vi "AlliGator Compute Pixel Phasor Array v3.vi"(6 "e^j w t_i Vector":csg[](array[numeric]), 7 "Time-Gated Reference Decay":cluster{"t Array":dbl[], "I Array":dbl[]}, 8 "Error In":errorcluster, 9 "t Array":sgl[](array[numeric]), 10 "Gate Images Stack (NxVxH)":sgl[][][](array[numeric]), 11 "Sum Image (V x H)":sgl[][](array[numeric])) -> (0 "Error Out":errorcluster, 1 "# Invalid Phasors":i32, 3 "Pixel Phasors Array (V x H)":csg[][](array[numeric]) format="%_3e", 4 "CPU (s)":dbl)   [LabVIEW 2021, in "AlliGator Phasor Plot.lvlib"]
doc: "Computes the phasor of all pixels using any user-selected decay pre-processing options."
uses:
  AlliGator Phasor Plot.lvlib
  AlliGator Settings List.ctl
  AlliGator Abort.vi
  <vilib>/Utility/error.llb/Error Cluster From Error Code.vi
  <vilib>/ErrorRing/Error Ring.xnode
  Time/Time.lvlib
  Phasor/Phasor.lvlib
  Graphs/XY Graph/XY Graph Add-Ons.lvlib
  AlliGator Decay Preprocessing.lvlib
  AlliGator Globals, Variables & Constants.lvlib
  AlliGator Settings.lvlib
  Error/Error.lvlib
  Utilities/Utilities.lvlib
panel:
  out "Local Error":errorcluster
  # "see the AlliGator License on the block diagram (Ctrl+E or Window:Show Block Diagram)"
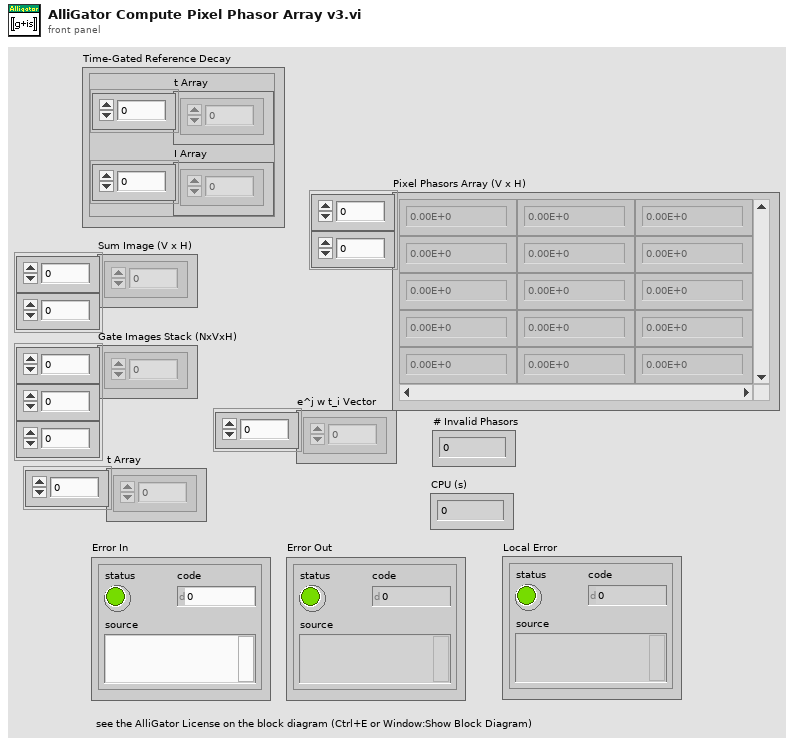
[diagram p1: front panel]
types:
  T1 = typedef "AlliGator Settings.lvlib/AlliGator Settings List.ctl" = enum16{"GUI:Visible Settings Tab", "GUI:Last Run Version", "Source Image:Use Image Histogram for Contrast", "Source Image:Low Count Pixels Rejection Options", "Source Image:High Count Pixels Rejection Options", "Source Image:Use Image Brightness", "Source Image:Blend Overlay with Image Background", "Source Image:Use Fixed ROI Diameter", "Source Image:ROI Diameter", "Source Image:ROI Center Color", "Source Image:Peak Threshold", "Source Image:Intensity Threshold", "Source Image:Image Binning Options", "Source Image:Image Smoothing Options", "Source Image:Image Histogram Active", "Source Image:Invert Binary Mask", "Source Image:Hot Pixel Removal", "Source Image:Overlay Analyzed ROI Center", "Source Image:Auto-Adjust Contrast", "Source Image:Histogram Lower Percentile", "Source Image:Histogram Upper Percentile", "Source Image:Save Source Image", "Source Image:Scale Bar Options", "Source Image:Image Resolution (Pixel Size)", "Source Image:Flatfield Correction", "Source Image:Show Dead Left Columns Correction", "Source Image:Dead Left Columns Correction", "Source Image:Image Pre-Processing Operations Order", "Source Image:Overlay ROI Median", "Source Image:Median Overlay Color", "Data Information:Gate Width", "Data Information:Nanotime Gate Separation", "Data Information:Macrotime Gate Separation", "Data Information:Gate Step", "Data Information:# Gates", "Data Information:Gate Image Exposure", "Data Information:Gate Image Integration", "Data Information:Gates to Skip", "Data Information:Gates to Keep", "Data Information:Define Gates to", "Data Information:Channel Name", "Data Information:Available Channel Names", "Data Information:Channel Arithmetic", "Data Information:Background File Subtraction", "Data Information:Background File", "Data Information:Background Scaling Factor", "Data Information:Background Pile-up Correction", "Data Information:Background Pixel Well Capacity", "Data Information:Laser Period", "Data Information:SYNC Period", "Data Information:Pile-up Correction", "Data Information:Pixel Well Capacity", "Data Information:Dataset Scaling Factor", "Fluorescence Decay_Decay Pre-Processing:Reverse Gates", "Fluorescence Decay_Decay Pre-Processing:Verbose Decay Pre-Processing", "Fluorescence Decay_Decay Pre-Processing:Use Decay Pre-Processing", "Fluorescence Decay_Decay Pre-Processing:Background Subtraction", "Fluorescence Decay_Decay Pre-Processing:Background Definition Range", "Fluorescence Decay_Decay Pre-Processing:Baseline Subtraction Method", "Fluorescence Decay_Decay Pre-Processing:Decay Pre-Processing Operations Order", "Fluorescence Decay_Decay Pre-Processing:Smoothing Parameter", "Fluorescence Decay_Decay Pre-Processing:Shift Decay", "Fluorescence Decay_Decay Pre-Processing:Decay Shift Parameters", "Fluorescence Decay_Decay Pre-Processing:Fold Decay", "Fluorescence Decay_Decay Pre-Processing:# Folds", "Fluorescence Decay_Decay Pre-Processing:1-Normalize Decay", "Fluorescence Decay_Decay Pre-Processing:[0-1]-Normalize Decay", "Fluorescence Decay_Decay Pre-Processing:Smoothen Decay", "Fluorescence Decay_Decay Pre-Processing:Extrapolate Decay", "Fluorescence Decay_Decay Pre-Processing:Use Periodicity", "Fluorescence Decay_Decay Pre-Processing:Use Cursors", "Fluorescence Decay_Decay Pre-Processing:Tail Fraction", "Fluorescence Decay_Decay Pre-Processing:Head Fraction", "Fluorescence Decay_Decay Pre-Processing:Additional Points", "Fluorescence Decay_Decay Pre-Processing:Straighten Decay", "Fluorescence Decay_Decay Pre-Processing:Constant Background", "Fluorescence Decay_Decay Pre-Processing:Pixel-Normalize Decay", "Fluorescence Decay_Advanced Analysis:Extract IRF instead of Decay", "Fluorescence Decay_Advanced Analysis:IRF Extraction Options", "Fluorescence Decay_Advanced Analysis:IRF Optimization Options", "Fluorescence Decay_Advanced Analysis:Square Pulse Options", "Fluorescence Decay_Advanced Analysis:IRF Order", "Fluorescence Decay_Advanced Analysis:IRF Time Constants", "Fluorescence Decay_Advanced Analysis:Wavelet Analysis Options", "Fluorescence Decay_Advanced Analysis:Average Lifetime Options", "Fluorescence Decay_Fit Options:Fit Options", "Fluorescence Decay_Fit Options:Use Legacy Fitting Approach", "Fluorescence Decay_Fit Options:Use Data Information Laser Period", "Fluorescence Decay_Fit Parameters:Displayed Fit Parameters", "Fluorescence Decay_Fit Parameters:Fit Parameter Constraints", "Fluorescence Decay_Fit Parameters:Export Tabulated Results", "Fluorescence Decay_Fit Parameters:MLE Baseline Offset Type", "Fluorescence Decay_Fit Parameters:MLE Baseline Offset", "Fluorescence Decay_Fit Parameters:Guess Parameter Names", "Fluorescence Decay_Fit Parameters:Guess Parameter Values", "Fluorescence Decay_Fit Parameters:Guess Parameters Options", "Fluorescence Decay_Styles:Show Last Decay Only", "Fluorescence Decay_Styles:Decay Graph Color Array", "Fluorescence Decay:Decay Graph Active", "Fluorescence Decay Statistics:Min Peak Value", "Fluorescence Decay Statistics:Reject Low Decay Peak Pixels", "Fluorescence Decay Statistics:Reject High Decay Peak Pixels", "Fluorescence Decay Statistics:Max Peak Value", "Time Traces:Use File Timestamp", "Time Traces:Time Step", "Time Traces:Use Intensity Correction File", "Time Traces:Intensity Correction File", "Phasor Plot:Phasor Plot Smoothing Options", "Phasor Plot:Phasor Plot Size", "Phasor Plot:Phasor Plot Graphics Options", "Phasor Plot:Cumulative Phasor Plot", "Phasor Plot:Use Phasor Brightness", "Phasor Plot:Blend Overlay with Phasor Background", "Phasor Plot:Save Phasor Plot", "Phasor Plot:Show References", "Phasor Plot:Phasor Ratio Decay Range", "Phasor Plot:Exponential Fading", "Phasor Plot:Phasor Ratio Reference Colors", "Phasor Plot:Reference Radius", "Phasor Plot:Show Color Map Vertices", "Phasor Plot:Phasor Plot Active", "Phasor Plot:Phasor Ratio Color Map Type", "Phasor Plot:Phasor Ratio Color Map", "Phasor Plot:Phasor Ratio Display Range", "Phasor Plot:Selected Image ROI(s)", "Phasor Plot:All Image ROIs", "Phasor Plot:Selected Phasor Plot ROI(s)", "Phasor Plot:All Phasor Plot ROIs", "Phasor Plot:Phasor Ratio Color-Coded Quantity", "Phasor Plot:Store Phasor Harmonics", "Phasor Plot:Draw Reference Segment", "Phasor Plot:User-Defined Quantity", "Phasor Graph:Phasor Frequency", "Phasor Graph:Phasor Ratio Type", "Phasor Graph:Pixel-level Phasor Computation", "Phasor Graph:Save Phasor Graph", "Phasor Graph:Phasor Graph Active", "Phasor Graph:Phasor SDV Options", "Phasor Calibration:Use Backup Calibration if needed", "Phasor Graph:Define Shortest Lifetime as", "Phasor Calibration:Backup Calibration Type", "Phasor Calibration:Calibration Type", "Phasor Calibration:Calibration Lifetime", "Phasor Calibration:Calibration Map Algorithm", "Single-Exponential Phasor Locus (SEPL):Gate Parameters", "Single-Exponential Phasor Locus (SEPL):User-defined Gate", "Single-Exponential Phasor Locus (SEPL):User-defined IRF", "Single-Exponential Phasor Locus (SEPL):Phasor Parameters", "Single-Exponential Phasor Locus (SEPL):Decay & IRF Parameters", "Single-Exponential Phasor Locus (SEPL):Display Parameters", "Lifetime Analysis:Decay Analysis Parameters", "Lifetime Analysis:Lifetime Map Active", "Plugins:Python Settings", "Miscellaneous:Verbose Mode", "Miscellaneous:Beep after Script", "Miscellaneous:Saved Image File Format", "Miscellaneous:Exported Gate Image Settings", "Miscellaneous:Include Loading in Timing", "Miscellaneous:Verbose Settings Mode", "Miscellaneous:Histogram Options", "Miscellaneous:Beep on Error", "Miscellaneous:# Logical Processors Used", "Miscellaneous:ROI Description Max Characters", "Miscellaneous:Verbose Error Mode", "Miscellaneous:Transparent Mask Color"}
  T2 = typedef "AlliGator Decay Analysis.lvlib/AlliGator Decay Preprocessing.lvlib/AlliGator Decay Preprocessing Options.ctl" = cluster{"Background Subtraction Parameters":T3, "Decay Preprocessing Parameters":T5, "Preprocessing Steps Order":string[]}
  T3 = typedef "AlliGator Decay Analysis.lvlib/AlliGator Decay Preprocessing.lvlib/AlliGator Background Subtraction Parameters.ctl" = cluster{"Background Definition Range":cluster{"Min Gate":dbl[unit], "Max Gate":dbl[unit]}, "Baseline Subtraction Method":T4, "Background Subtraction?":bool, "Background File":path, "Background Constant":dbl, "Background Scaling Factor":dbl, "Background Pile-up Correction":bool, "Background Pixel Well Capacity":u32}
  T4 = typedef "AlliGator Decay Analysis.lvlib/AlliGator Decay Preprocessing.lvlib/AlliGator Baseline Subtraction Method.ctl" = enum16{"Mean", "Min", "Square Gated Single-Exponential", "File", "Constant"}
  T5 = typedef "AlliGator Decay Analysis.lvlib/AlliGator Decay Preprocessing.lvlib/AlliGator Decay Preprocessing Parameters.ctl" = cluster{"Background Subtraction":bool, "Straighten Decay":bool, "Reverse Gates":bool, "1-Normalized Decay":bool, "Smoothen Decay":bool, "Smoothing Parameter":dbl, "Shift Decay":bool, "Decay Shift Parameters":T6, "Extrapolate Decay":bool, "Additional Points":u32, "Head Fraction":dbl, "Pixel-Normalize Decay":bool, "Use Periodicity":bool, "Use Cursors":bool, "Tail Fraction":dbl, "Use Decay Pre-Processing":bool, "Fold Decay":bool, "# Folds":u32, "[0-1]-Normalized Decay":bool}
  T6 = typedef "XY Graph Add-Ons.lvlib/XY Graph Plot Shift Parameters.ctl" = cluster{"Type":T7, "Shift":dbl[unit], "Threshold":dbl, "Rotate":bool}
  T7 = typedef "XY Graph Add-Ons.lvlib/XY Graph Plot Shift Method.ctl" = enum16{"Default", "CFD", "Threshold", "Cross-Correlation"}
  T8 = cluster{"Min Gate":dbl[unit], "Max Gate":dbl[unit]}
  T9 = cluster{"t Axis":dbl[], "ROI Intensity Array in":dbl[]}
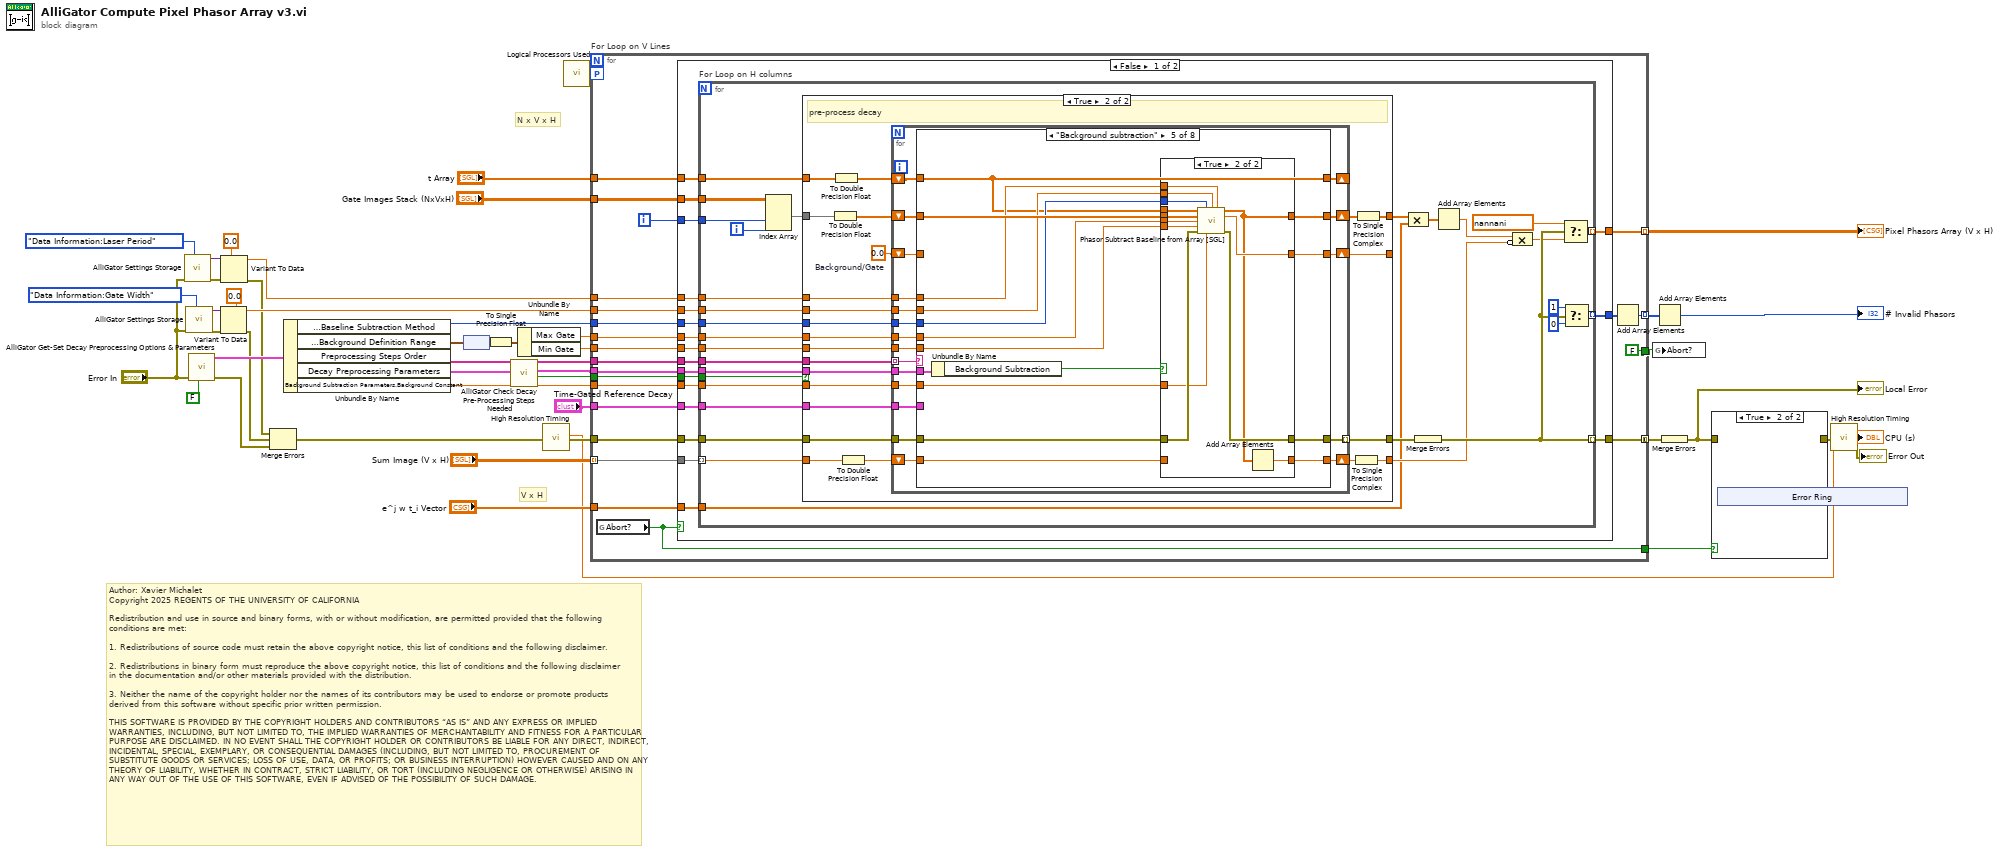
[diagram p0: block diagram]
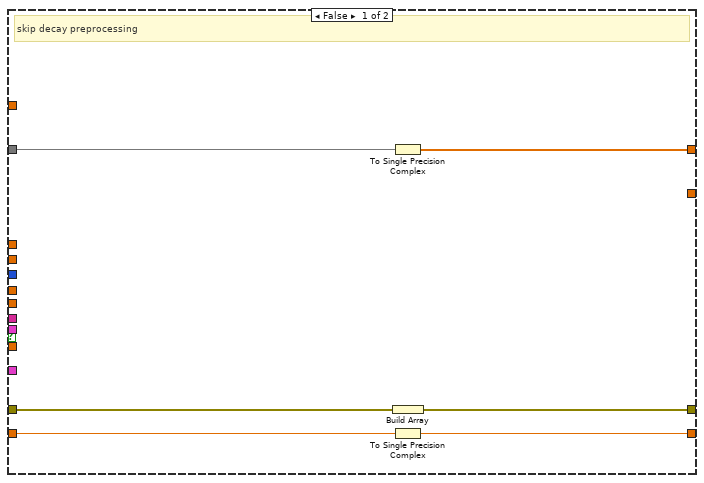
[diagram p2: hidden frame]
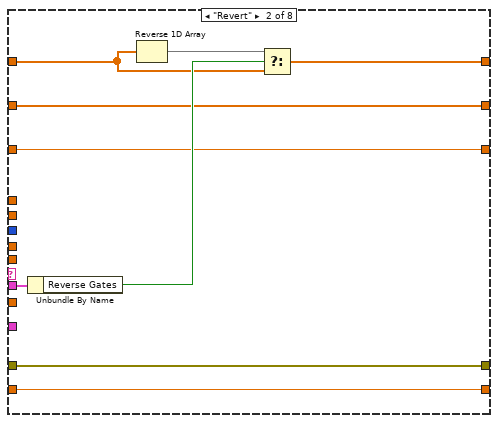
[diagram p4: hidden frame]
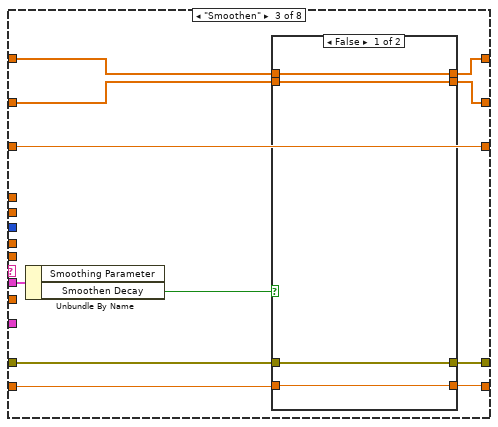
[diagram p5: hidden frame]
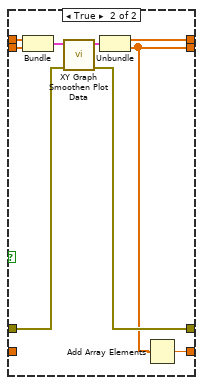
[diagram p6: hidden frame]
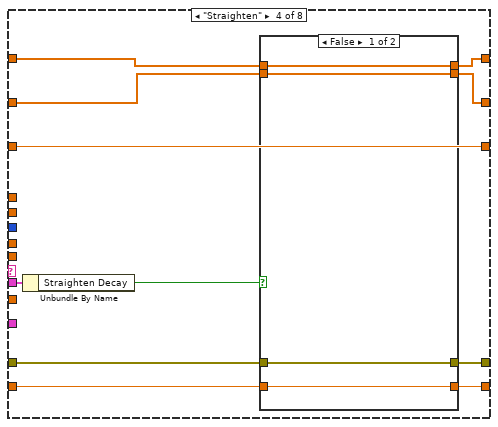
[diagram p7: hidden frame]
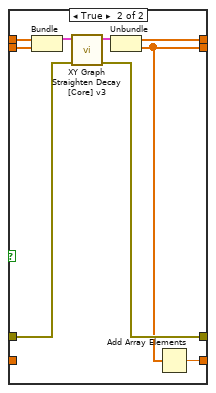
[diagram p8: hidden frame]
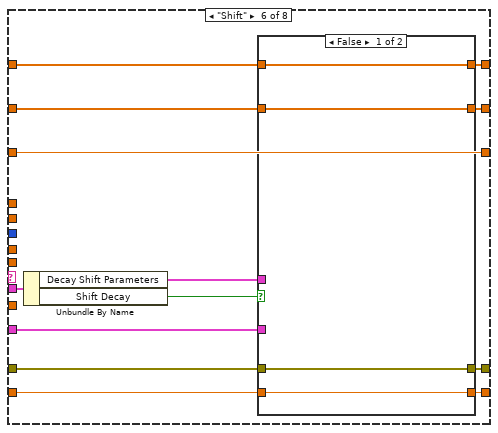
[diagram p10: hidden frame]
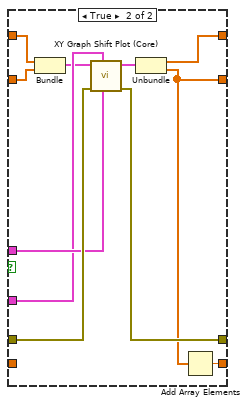
[diagram p11: hidden frame]
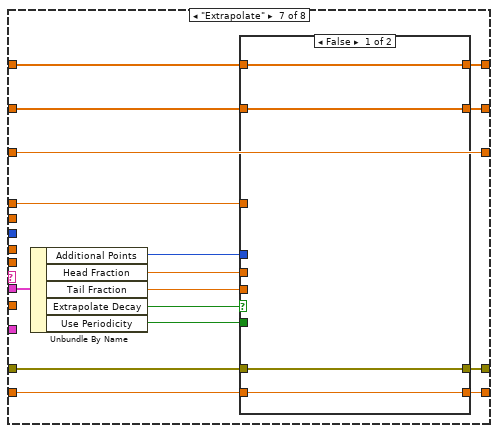
[diagram p12: hidden frame]
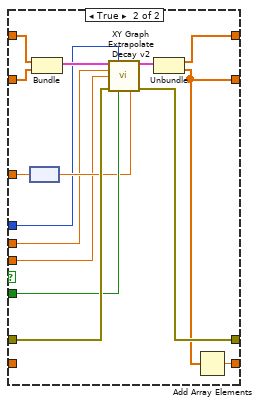
[diagram p13: hidden frame]
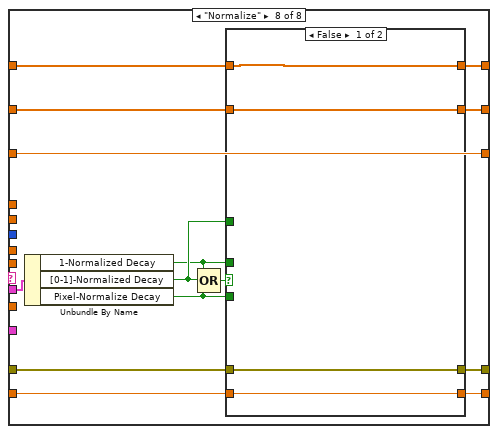
[diagram p14: hidden frame]
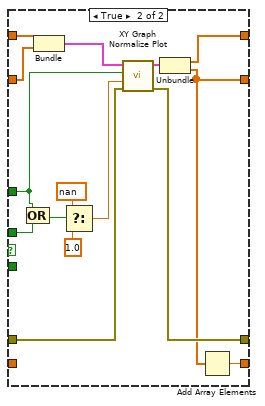
[diagram p15: hidden frame]
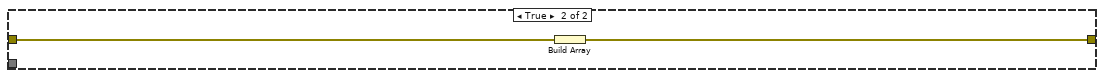
[diagram p16: hidden frame]
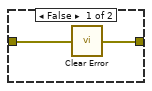
[diagram p17: hidden frame]
diagram:
  # "Author: Xavier Michalet\nCopyright 2025 REGENTS OF THE UNIVERSITY OF CALIFORNIA\n\nRedistribution and use in source and binary forms, with or without modification, are permitted provided that the following conditions are met:\n\n1. Redistributions of source code must retain the above copyright notice, this list of conditions and the following disclaimer.\n\n2. Redistributions in binary form must reproduce the above copyright notice, this list of conditions and the following disclaimer in the documentation and/or other materials provided with the distribution.\n\n3. Neither the name of the copyright holder nor the names of its contributors may be used to endorse or promote products derived from this software without specific prior written permission.\n\nTHIS SOFTWARE IS PROVIDED BY THE COPYRIGHT HOLDERS AND CONTRIBUTORS “AS IS” AND ANY EXPRESS OR IMPLIED WARRANTIES, INCLUDING, BUT NOT LIMITED TO, THE IMPLIED WARRANTIES OF MERCHANTABILITY AND FITNESS FOR A PARTICULAR PURPOSE ARE DISCLAIMED. IN NO EVENT SHALL THE COPYRIGHT HOLDER OR CONTRIBUTORS BE LIABLE FOR ANY DIRECT, INDIRECT, INCIDENTAL, SPECIAL, EXEMPLARY, OR CONSEQUENTIAL DAMAGES (INCLUDING, BUT NOT LIMITED TO, PROCUREMENT OF SUBSTITUTE GOODS OR SERVICES; LOSS OF USE, DATA, OR PROFITS; OR BUSINESS INTERRUPTION) HOWEVER CAUSED AND ON ANY THEORY OF LIABILITY, WHETHER IN CONTRACT, STRICT LIABILITY, OR TORT (INCLUDING NEGLIGENCE OR OTHERWISE) ARISING IN ANY WAY OUT OF THE USE OF THIS SOFTWARE, EVEN IF ADVISED OF THE POSSIBILITY OF SUCH DAMAGE."
  # "V x H"
  # "N x V x H"
  n1 = call "AlliGator Settings Storage.vi"("AlliGator Settings List"=AlliGator_Settings_List."Data Information:Laser Period", "Error In"="Error In") -> ("Error Out"=w24:errorcluster, "Variant Data out"=w25:variant)  [unwired: 8 in]
  n2 = call "AlliGator Settings Storage.vi"("AlliGator Settings List"=AlliGator_Settings_List."Data Information:Gate Width", "Error In"="Error In") -> ("Error Out"=w14:errorcluster, "Variant Data out"=w23:variant)  [unwired: 8 in]
  n3 = call "AlliGator Get-Set Decay Preprocessing Options & Parameters.vi"("Get (F)/Set"=FALSE, "error in (no error)"="Error In") -> ("error out"=w35:errorcluster, "Decay Preprocessing Options & Parameters out"=w29:T2)  [unwired: 8 in]
  n4 = Variant To Data(error in=w14, type=dbl[unit] 0.0 ("Laser Period"), Variant=w23) -> (data=w18:dbl[unit], error out=w16:errorcluster)
  n5 = Variant To Data(error in=w24, type=dbl[unit] 0.0 ("Laser Period"), Variant=w25) -> (data=w19:dbl[unit], error out=w15:errorcluster)
  n6 = Merge Errors(w15, w16, w35) -> (w17:errorcluster)
  n7 = Unbundle By Name(w29) -> ("Background Subtraction Parameters.Baseline Subtraction Method"=w28:T4, "Background Subtraction Parameters.Background Definition Range"=w27:T8, "Preprocessing Steps Order"=w7:string[], "Decay Preprocessing Parameters"=w6:T5, "Background Subtraction Parameters.Background Constant"=w8:dbl)
  n8 = node(w27) -> (w37:cluster{"Min Gate":dbl, "Max Gate":dbl})
  n9 = To Single Precision Float(number=w37) -> (single precision float=w36:cluster{"Min Gate":sgl, "Max Gate":sgl})
  n10 = call "AlliGator Check Decay Pre-Processing Steps Needed.vi"("Decay Preprocessing Parameters"=w6, "Preprocessing Steps Order in"=w7) -> ("Preprocessing needed?"=w3:bool, "Decay Preprocessing Parameters (dup)"=w4:T5, "Preprocessing Steps Order out"=w5:string[])  [unwired: 7 in]
  n11 = Unbundle By Name(w36) -> ("Max Gate"=w45:sgl, "Min Gate"=w44:sgl)
  n12 = call "High Resolution Timing.vi"("Error In"=w17) -> ("elapsed (relative) seconds"=w31:dbl, "Error Out"=w34:errorcluster)  [unwired: 16 in, 1 out]
  n13 = call "Logical Processors Used.vi"() -> ("# Logical Processor Used"=w1:i32)  [unwired: 6 in]
  n14 = for "For Loop on V Lines" {
    tunnel: "Gate Images Stack (NxVxH)" -> [w69]
    tunnel: "e^j w t_i Vector" -> [w68]
    tunnel: "Sum Image (V x H)" -> [w67] mode=indexing
    tunnel: [w65] -> w43 mode=indexing
    tunnel: "t Array" -> [w64]
    tunnel: w45 -> [w63]
    tunnel: w44 -> [w62]
    tunnel: w28 -> [w61]
    tunnel: w18 -> [w60]
    tunnel: w19 -> [w59]
    tunnel: [w50] -> w38
    tunnel: w34 -> [w58]
    tunnel: [w57] -> w33 mode=concatenating
    tunnel: "Time-Gated Reference Decay" -> [w56]
    tunnel: w5 -> [w55]
    tunnel: w4 -> [w54]
    workers-P: w1 -> [_]
    tunnel: [FALSE ("Abort?")] -> w13
    tunnel: [w51] -> w11 mode=indexing
    tunnel: w8 -> [w49]
    tunnel: w3 -> [w48]
    i -> [w66]
    n15 = global read "AlliGator Abort.vi" "Abort?"() -> (w50:bool)
    n16 = case shown="False" w50 {
      tunnel: w69 -> [w88 _]
      tunnel: w68 -> [w87 _]
      tunnel: w67 -> [w86 _]
      tunnel: w66 -> [w85 _]
      tunnel: [w84 _] -> w65
      tunnel: w64 -> [w83 _]
      tunnel: w63 -> [w82 _]
      tunnel: w62 -> [w81 _]
      tunnel: w61 -> [w80 _]
      tunnel: w60 -> [w79 _]
      tunnel: w59 -> [w78 _]
      tunnel: w58 -> [w77 w357]
      tunnel: [w76 w356] -> w57
      tunnel: w56 -> [w75 _]
      tunnel: w55 -> [w74 _]
      tunnel: w54 -> [w73 _]
      tunnel: [w72 _] -> w52
      tunnel: w49 -> [w71 _]
      tunnel: w48 -> [w70 _]
      frame False {
        n17 = for "For Loop on H columns" {
          tunnel: w88 -> [w118]
          tunnel: w87 -> [w90]
          tunnel: w85 -> [w113]
          tunnel: w86 -> [w92] mode=indexing
          tunnel: [w100] -> w84 mode=indexing
          tunnel: w83 -> [w106]
          tunnel: w82 -> [w111]
          tunnel: w81 -> [w110]
          tunnel: w80 -> [w112]
          tunnel: w79 -> [w109]
          tunnel: w78 -> [w108]
          tunnel: w77 -> [w105]
          tunnel: [w98] -> w76 mode=indexing
          tunnel: w75 -> [w103]
          tunnel: w74 -> [w102]
          tunnel: w73 -> [w101]
          tunnel: [w95] -> w72 mode=indexing
          tunnel: w71 -> [w94]
          tunnel: w70 -> [w93]
          i -> [w114]
          n18 = Index Array(array=w118, index (dim 1)=w113, index (dim 2)=w114) -> (element=w115:sgl[])  [unwired: 1 in]
          n19 = case shown="True" w93 {
            tunnel: w115 -> [w124 w147]
            tunnel: w112 -> [_ w146]
            tunnel: w111 -> [_ w145]
            tunnel: w110 -> [_ w144]
            tunnel: [_ w143] -> _
            tunnel: w109 -> [_ w142]
            tunnel: w108 -> [_ w141]
            tunnel: [w120 w126] -> w107
            tunnel: w106 -> [_ w138]
            tunnel: w105 -> [w123 w137]
            tunnel: [w122 w136] -> w104
            tunnel: w103 -> [_ w135]
            tunnel: w102 -> [_ w134]
            tunnel: w101 -> [_ w133]
            tunnel: w94 -> [_ w132]
            tunnel: w92 -> [w121 w131]
            tunnel: [w119 w125] -> w91
            frame False {
              # "skip decay preprocessing"
              n20 = To Single Precision Complex(1:w124) -> (0:w120:csg[])
              n21 = Build Array(w123) -> (w122:errorcluster[])
              n22 = To Single Precision Complex(1:w121) -> (0:w119:csg)
            }
            frame True {
              w140 = 0.0  # Background/Gate
              # "pre-process decay"
              n23 = To Double Precision Float(number=w147) -> (double precision float=w128:dbl[])
              n24 = To Double Precision Float(number=w138) -> (double precision float=w129:dbl[])
              n25 = To Double Precision Float(number=w131) -> (double precision float=w127:dbl)
              n26 = for {
                tunnel: w146 -> [w165]
                tunnel: w145 -> [w164]
                tunnel: w144 -> [w163]
                tunnel: w142 -> [w161]
                tunnel: w141 -> [w160]
                shift-right: [w162] -> w143
                shift-left: w140 -> [w159]
                shift-right: [w158] -> w139
                shift-left: w128 -> [w166]
                shift-right: [w156] -> _
                shift-left: w129 -> [w157]
                tunnel: w137 -> [w155]
                tunnel: [w154] -> w136 mode=indexing
                tunnel: w135 -> [w153]
                tunnel: w134 -> [w152] mode=indexing
                tunnel: w133 -> [w151]
                tunnel: w132 -> [w150]
                shift-right: [w148] -> w130
                shift-left: w127 -> [w149]
                n27 = case shown="\"Background subtraction\"" w152 {
                  tunnel: w157 -> [w170 w179 w188 w213 w235 w267 w299 w333]
                  tunnel: w166 -> [w169 w175 w189 w212 w244 w265 w297 w331]
                  tunnel: [w169 w175 w186 w210 w243 w264 w296 w330] -> w158
                  tunnel: w165 -> [_ _ _ _ w242 _ _ _]
                  tunnel: w164 -> [_ _ _ _ w241 _ _ _]
                  tunnel: w163 -> [_ _ _ _ w240 _ _ _]
                  tunnel: [w171 w177 w191 w215 w239 w273 w303 w336] -> w162
                  tunnel: w161 -> [_ _ _ _ w238 _ _ _]
                  tunnel: w160 -> [_ _ _ _ w237 _ w291 _]
                  tunnel: w159 -> [w171 w177 w191 w215 _ w273 w303 w336]
                  tunnel: [w170 w176 w187 w211 w235 w266 w298 w332] -> w156
                  tunnel: w155 -> [w168 w174 w185 w209 w234 w269 w301 w335]
                  tunnel: [w168 w174 w184 w208 w233 w268 w300 w334] -> w154
                  tunnel: w153 -> [_ _ _ _ _ w270 _ _]
                  tunnel: w151 -> [_ w173 w183 w207 w232 w263 w294 w329]
                  tunnel: w150 -> [_ _ _ _ w231 _ _ _]
                  tunnel: w149 -> [w167 w172 w182 w206 w230 w261 w289 w327]
                  tunnel: [w167 w172 w181 w205 w229 w262 w290 w326] -> w148
                  frame Default {
                  }
                  frame "Revert" {
                    n28 = Unbundle By Name(w173) -> ("Reverse Gates"=w180:bool)
                    n29 = Reverse 1D Array(array=w179) -> (reversed array=w178:dbl[])
                    n30 = Select(t=w178, s=w180, f=w179) -> (s? t:f=w176:dbl[])
                  }
                  frame "Smoothen" {
                    n31 = Unbundle By Name(w183) -> ("Smoothen Decay"=w190:bool)  [unwired: 1 out]
                    n32 = case shown="False" w190 {
                      tunnel: w188 -> [w195 w204]
                      tunnel: w189 -> [w194 w203]
                      tunnel: [w195 w200] -> w187
                      tunnel: [w194 w197] -> w186
                      tunnel: w185 -> [w193 w199]
                      tunnel: [w193 w198] -> w184
                      tunnel: w182 -> [w192 _]
                      tunnel: [w192 w196] -> w181
                      frame False {
                      }
                      frame True {
                        n33 = Bundle(w204, w203) -> (w202:cluster{dbl[], dbl[]})  [unwired: 1 in]
                        n34 = call "XY Graph Smoothen Plot Data.vi"("Error In"=w199, "Plot"=w202) -> ("error out"=w198:errorcluster, "Cubic Splined Plot"=w201:cluster{"X Array":dbl[], "Y Array":dbl[]})  [unwired: 8 in]
                        n35 = Unbundle(w201) -> ("X Array"=w200:dbl[], "Y Array"=w197:dbl[])
                        n36 = Add Array Elements(numeric array=w197) -> (sum=w196:dbl)
                      }
                    }
                  }
                  frame "Straighten" {
                    n37 = Unbundle By Name(w207) -> ("Straighten Decay"=w214:bool)
                    n38 = case shown="False" w214 {
                      tunnel: w213 -> [w219 w228]
                      tunnel: w212 -> [w218 w227]
                      tunnel: [w219 w224] -> w211
                      tunnel: [w218 w221] -> w210
                      tunnel: w209 -> [w217 w223]
                      tunnel: [w217 w222] -> w208
                      tunnel: w206 -> [w216 _]
                      tunnel: [w216 w220] -> w205
                      frame False {
                      }
                      frame True {
                        n39 = Bundle(w228, w227) -> (w226:cluster{dbl[], dbl[]})  [unwired: 1 in]
                        n40 = call "XY Graph Straighten Decay [Core] v3.vi"("Error In"=w223, "Plot in"=w226) -> ("error out"=w222:errorcluster, "Plot out"=w225:cluster{"X Array":dbl[], "Y Array":dbl[]})  [unwired: 7 in, 1 out]
                        n41 = Unbundle(w225) -> ("X Array"=w224:dbl[], "Y Array"=w221:dbl[])
                        n42 = Add Array Elements(numeric array=w221) -> (sum=w220:dbl)
                      }
                    }
                  }
                  frame "Background subtraction" {
                    n43 = Unbundle By Name(w232) -> ("Background Subtraction"=w236:bool)
                    n44 = case shown="True" w236 {
                      tunnel: w235 -> [_ w260]
                      tunnel: w244 -> [w247 w259]
                      tunnel: [w247 w249] -> w243
                      tunnel: w242 -> [_ w258]
                      tunnel: w241 -> [_ w257]
                      tunnel: w240 -> [_ w256]
                      tunnel: [_ w255] -> w239
                      tunnel: w238 -> [_ w254]
                      tunnel: w237 -> [_ w253]
                      tunnel: w234 -> [w246 w252]
                      tunnel: [w246 w251] -> w233
                      tunnel: w231 -> [_ w250]
                      tunnel: w230 -> [w245 _]
                      tunnel: [w245 w248] -> w229
                      frame False {
                      }
                      frame True {
                        n45 = call "Phasor Subtract Baseline from Array [SGL].vi"("X Array"=w260, "Method (Min)"=w258, "Gate Duration"=w254, "Laser Period"=w253, "Y Array"=w259, "Max X"=w257, "Min X"=w256, "Error In"=w252, "Background Constant"=w250) -> ("Bkgd-subtracted Y Array"=w249:sgl[], "Background/Gate"=w255:sgl, "Error Out"=w251:errorcluster)  [unwired: 1 in, 3 out]
                        n46 = Add Array Elements(numeric array=w249) -> (sum=w248:sgl)
                      }
                    }
                  }
                  frame "Shift" {
                    n47 = Unbundle By Name(w263) -> ("Decay Shift Parameters"=w271:T6, "Shift Decay"=w272:bool)
                    n48 = case shown="False" w272 {
                      tunnel: w271 -> [_ w286]
                      tunnel: w270 -> [_ w285]
                      tunnel: w269 -> [w277 w288]
                      tunnel: [w277 w287] -> w268
                      tunnel: w267 -> [w276 w284]
                      tunnel: [w276 w280] -> w266
                      tunnel: w265 -> [w275 w283]
                      tunnel: [w275 w279] -> w264
                      tunnel: [w274 w278] -> w262
                      tunnel: w261 -> [w274 _]
                      frame False {
                      }
                      frame True {
                        n49 = Bundle(w284, w283) -> (w282:cluster{dbl[], dbl[]})  [unwired: 1 in]
                        n50 = call "XY Graph Shift Plot (Core).vi"("Plot Shift Parameters"=w286, "Time-Gated Reference Decay"=w285, "error in (no error)"=w288, "Decay in"=w282) -> ("error out"=w287:errorcluster, "Decay out"=w281:T9)  [unwired: 5 in, 1 out]
                        n51 = Unbundle(w281) -> ("t Axis"=w280:dbl[], "ROI Intensity Array in"=w279:dbl[])
                        n52 = Add Array Elements(numeric array=w279) -> (sum=w278:dbl)
                      }
                    }
                  }
                  frame "Extrapolate" {
                    n53 = Unbundle By Name(w294) -> ("Additional Points"=w295:u32, "Head Fraction"=w292:dbl, "Extrapolate Decay"=w302:bool, "Use Periodicity"=w293:bool)  [unwired: 1 out]
                    n54 = case shown="False" w302 {
                      tunnel: w301 -> [w307 w322]
                      tunnel: [w307 w321] -> w300
                      tunnel: w299 -> [w306 w320]
                      tunnel: [w306 w316] -> w298
                      tunnel: w297 -> [w305 w319]
                      tunnel: [w305 w309] -> w296
                      tunnel: w292 -> [_ w311]
                      tunnel: w295 -> [_ w312]
                      tunnel: w293 -> [_ w315]
                      tunnel: w291 -> [_ w314]
                      tunnel: w292 -> [_ w310]
                      tunnel: [w304 w308] -> w290
                      tunnel: w289 -> [w304 _]
                      frame False {
                      }
                      frame True {
                        n55 = node(w314) -> (w313:dbl)
                        n56 = Bundle(w320, w319) -> (w318:cluster{dbl[], dbl[]})  [unwired: 1 in]
                        n57 = call "XY Graph Extrapolate Decay v2.vi"("Plot in"=w318, "# Additional Points (-1: to Period)"=w312, "Head Fraction"=w310, "Tail Fraction"=w311, "Error In"=w322, "Periodic Decay"=w315, "Period"=w313) -> ("Plot out"=w317:cluster{"X Array":dbl[], "Y Array":dbl[]}, "error out"=w321:errorcluster)  [unwired: 3 in, 4 out]
                        n58 = Unbundle(w317) -> ("X Array"=w316:dbl[], "Y Array"=w309:dbl[])
                        n59 = Add Array Elements(numeric array=w309) -> (sum=w308:dbl)
                      }
                    }
                  }
                  frame "Normalize" {
                    n60 = Unbundle By Name(w329) -> ("1-Normalized Decay"=w323:bool, "[0-1]-Normalized Decay"=w325:bool, "Pixel-Normalize Decay"=w324:bool)
                    n61 = Compound Arithmetic op=OR(w323, w325, w324) -> (w328:bool)
                    n62 = case shown="False" w328 {
                      tunnel: w335 -> [w340 w355]
                      tunnel: [w340 w354] -> w334
                      tunnel: w333 -> [w338 w353]
                      tunnel: [w338 w349] -> w332
                      tunnel: w331 -> [w339 w352]
                      tunnel: [w339 w345] -> w330
                      tunnel: w327 -> [w337 _]
                      tunnel: [w337 w344] -> w326
                      tunnel: w325 -> [_ w343]
                      tunnel: w324 -> [_ _]
                      tunnel: w323 -> [_ w342]
                      frame False {
                      }
                      frame True {
                        n63 = Compound Arithmetic op=OR(w343, w342) -> (w341:bool)
                        n64 = Bundle(w353, w352) -> (w351:cluster{dbl[], dbl[]})  [unwired: 1 in]
                        n65 = Select(t=nan ("Normalization Factor"), s=w341, f=1.0) -> (s? t:f=w346:dbl)
                        n66 = call "XY Graph Normalize Plot.vi"("Error In"=w355, "Normalization Factor (Max *)"=w346, "Subtract Baseline? (No)"=w343, "Plot in"=w351) -> ("Error Out"=w354:errorcluster, "Plot out"=w350:cluster{"X Array":dbl[], "Y Array":dbl[]})  [unwired: 6 in]
                        n67 = Unbundle(w350) -> ("X Array"=w349:dbl[], "Y Array"=w345:dbl[])
                        n68 = Add Array Elements(numeric array=w345) -> (sum=w344:dbl)
                      }
                    }
                  }
                }
              }
              n69 = To Single Precision Complex(1:w130) -> (0:w125:csg)
              n70 = To Single Precision Complex(1:w139) -> (0:w126:csg[])
            }
          }
          n71 = Compound Arithmetic op=MULTIPLY(w107, w90) -> (w117:csg[])
          n72 = Merge Errors(w104) -> (w98:errorcluster)
          n73 = Add Array Elements(numeric array=w117) -> (sum=w116:csg)
          n74 = Compound Arithmetic op=MULTIPLY(w116, invert w91) -> (w89:csg)
          n75 = Select(t=csg nan+nani, s=w98, f=w89) -> (s? t:f=w100:csg)
          n76 = Select(t=1, s=w98, f=0) -> (s? t:f=w95:i32)
        }
      }
      frame True {
        n77 = Build Array(w357) -> (w356:errorcluster[])
      }
    }
    n78 = Add Array Elements(numeric array=w52) -> (sum=w51:i32)
  }
  "Pixel Phasors Array (V x H)" <- w43
  n79 = global write "AlliGator Abort.vi" "Abort?"(w13) -> ()
  n80 = Add Array Elements(numeric array=w11) -> (sum=→"# Invalid Phasors":i32)
  n81 = Merge Errors(w33) -> (w9:errorcluster)
  "Local Error" <- w9
  n82 = case shown="True" w38 {
    tunnel: [w358 w360] -> w32
    tunnel: w9 -> [w359 _]
    frame False {
      n83 = call "Clear Error.vi"("Error In"=w359) -> ("no Error Out"=w358:errorcluster)  [unwired: 8 in]
    }
    frame True {
      n84 = xnode "Error Ring"() -> ("error out"=w360:errorcluster)
    }
  }
  n85 = call "High Resolution Timing.vi"("relative seconds (NaN)"=w31, "Error In"=w32) -> ("elapsed (relative) seconds"=→"CPU (s)":dbl, "Error Out"=→"Error Out":errorcluster)  [unwired: 15 in, 1 out]
